vi "Check_Roadblock.vi"(9 "Posi_Roadblock":dbl[][](array[numeric]), 11 "New Posi":dbl[](array[numeric])) -> (1 "Hinderance":bool, 3 "Hinderance posi":dbl[](array[numeric]))   [LabVIEW 2020]
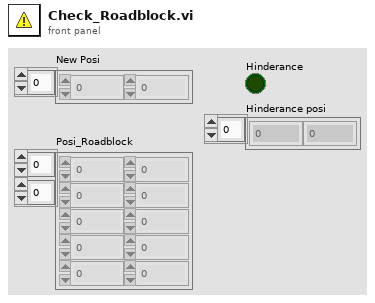
[diagram p1: front panel]
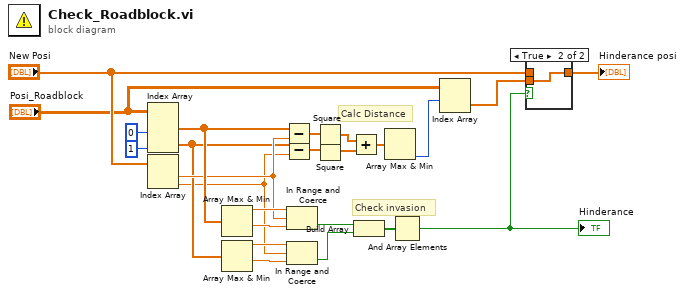
[diagram p0: block diagram]
diagram:
  (unwired) 0 ("disabled index (col)")
  (unwired) 0 ("disabled index (col)")
  (unwired) 0 ("disabled index (col)")
  # "Check invasion"
  # "Calc Distance"
  n1 = Index Array(array="Posi_Roadblock", index (col) #1=0 ("disabled index (col)"), index (col) #2=1 ("index (col)")) -> (element #1=w14:dbl[], element #2=w12:dbl[])  [unwired: 2 in]
  n2 = Index Array(array="New Posi") -> (element #1=w13:dbl, element #2=w11:dbl)  [unwired: 2 in]
  n3 = Array Max & Min(array=w14) -> (max value=w22:dbl, min value=w21:dbl)  [unwired: 2 out]
  n4 = Array Max & Min(array=w12) -> (max value=w20:dbl, min value=w19:dbl)  [unwired: 2 out]
  n5 = Subtract(x=w14, y=w13) -> (x-y=w10:dbl[])
  n6 = Subtract(x=w12, y=w11) -> (x-y=w9:dbl[])
  n7 = In Range and Coerce(upper limit=w22, x=w13, lower limit=w21) -> (In Range?=w18:bool)  [unwired: 1 out]
  n8 = In Range and Coerce(upper limit=w20, x=w11, lower limit=w19) -> (In Range?=w17:bool)  [unwired: 1 out]
  n9 = Square(x=w10) -> (x^2=w8:dbl[])
  n10 = Square(x=w9) -> (x^2=w7:dbl[])
  n11 = Add(x=w8, y=w7) -> (x+y=w6:dbl[])
  n12 = Build Array(w18, w17) -> (w16:bool[])
  n13 = Array Max & Min(array=w6) -> (min index (indices)=w5:i32)  [unwired: 3 out]
  n14 = And Array Elements(Boolean array=w16) -> (logical AND=w15:bool)
  "Hinderance" <- w15
  n15 = Index Array(array="Posi_Roadblock", index (row)=w5) -> (element=w4:dbl[])  [unwired: 1 in]
  n16 = case shown="TRUE" w15 {
    tunnel: w4 -> [_ w26]
    tunnel: [w25 w26] -> w3
    tunnel: "New Posi" -> [w25 _]
    frame False {
    }
    frame True {
    }
  }
  "Hinderance posi" <- w3
